vi "Process.vi"(8 "error in (no error)":errorcluster, 11 "ATS9462 Class in":refnum<class "ATS9462 Class.lvclass">) -> (0 "error out":errorcluster, 3 "ATS9462 Class out":refnum<class "ATS9462 Class.lvclass">)   [LabVIEW 2014, in "ATS9462 Class.lvclass"]
uses:
  ATS9462 Class.lvclass
  DAQ Class.lvclass
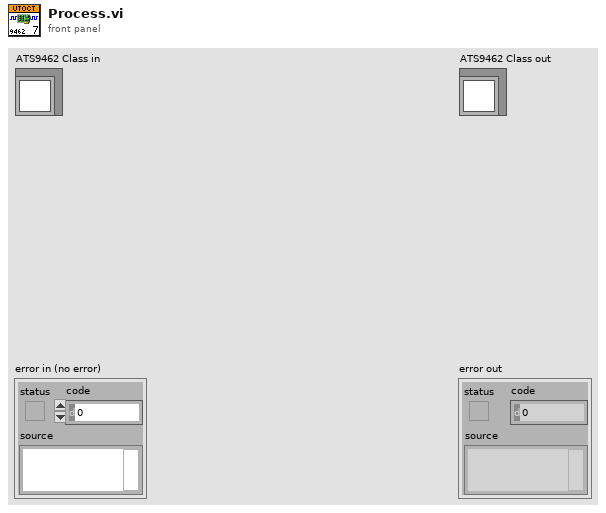
[diagram p1: front panel]
types:
  T1 = typedef "DAQ Class.lvclass/DAQ Modes.ctl" = enum16{"Real Time", "Save Data"}
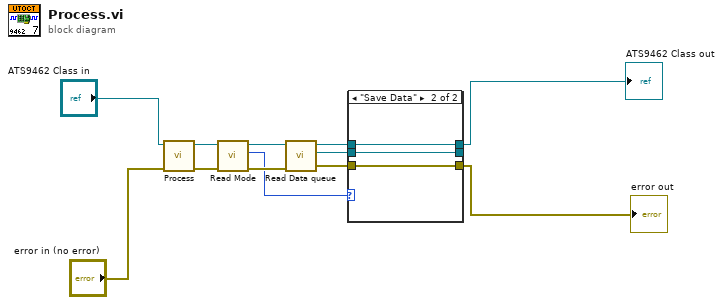
[diagram p0: block diagram]
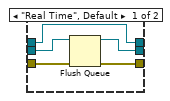
[diagram p2: hidden frame]
diagram:
  n1 = call-parent "Process.vi"("error in (no error)"="error in (no error)", "DAQ Class in"="ATS9462 Class in") -> ("error out"=w10:errorcluster, "DAQ Class out"=w9:refnum<class "ATS9462 Class.lvclass">)  [unwired: 8 in]
  n2 = call-dynamic "Read Mode.vi"("error in (no error)"=w10, "DAQ Class in"=w9) -> ("error out"=w8:errorcluster, "Mode"=w7:T1, "DAQ Class out"=w6:refnum<class "ATS9462 Class.lvclass">)  [unwired: 7 in]
  n3 = call-dynamic "Read Data queue.vi"("error in (no error)"=w8, "DAQ Class in"=w6) -> ("error out"=w5:errorcluster, "Data queue"=w4:refnum<queue>, "DAQ Class out"=w3:refnum<class "ATS9462 Class.lvclass">)  [unwired: 7 in]
  n4 = case shown="\"Save Data\"" w7 {
    tunnel: w5 -> [w17 w18]
    tunnel: w4 -> [w16 w19]
    tunnel: [w15 w19] -> _
    tunnel: [w14 w18] -> w2
    tunnel: w3 -> [w13 w20]
    tunnel: [w13 w20] -> w1
    frame "Real Time", Default {
      n5 = Flush Queue(queue=w16, error in (no error)=w17) -> (queue out=w15:refnum<queue>, error out=w14:errorcluster)  [unwired: 1 out]
    }
    frame "Save Data" {
    }
  }
  "error out" <- w2
  "ATS9462 Class out" <- w1
